vi "lvpeak_save_config.vi"(8 "error in (no error)":errorcluster, 10 "Path":path, 11 "camera_id":u64) -> (0 "error out":errorcluster)   [LabVIEW 2024, in "Vision.lvlib"]
uses:
  Vision.lvlib
  bin/LVPeak.dll
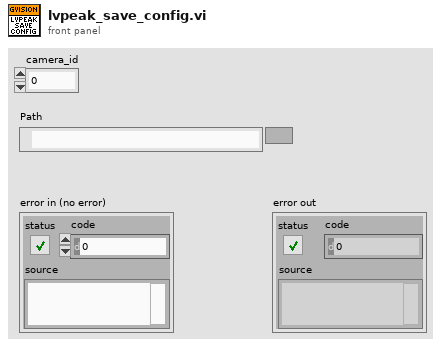
[diagram p1: front panel]
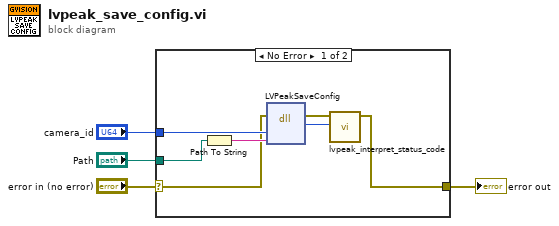
[diagram p0: block diagram]
diagram:
  n1 = case shown="No Error" "error in (no error)" {
    selector: "error in (no error)" -> [w6 w12]
    tunnel: [w5 w12] -> w3
    tunnel: "camera_id" -> [w9 _]
    tunnel: "Path" -> [w7 _]
    frame No Error {
      n2 = Path To String(path=w7) -> (string=w8:string)
      n3 = dll-call lib="C:/Users/cfang/Desktop/nebraska-silicon-lab/pixel-gantry-control/Gantry/Shared Components/bin/LVPeak.dll" fn="LVPeakSaveConfig"(error in=w6, "camera_id"=w9, "filename"=w8) -> (error out=w11:errorcluster, "return type"=w10:i32)  [unwired: 4 in, 1 out]
      n4 = call "lvpeak_interpret_status_code.vi"("status_code"=w10, "error in (no error)"=w11) -> ("error out"=w5:errorcluster)  [unwired: 9 in]
    }
    frame Error {
    }
  }
  "error out" <- w3
